vi "GetC.vi"(8 "L1":dbl, 9 "L":dbl, 10 "m":dbl, 11 "q":dbl[](array[numeric])) -> (2 "C":T1)   [LabVIEW 2019]
uses:
  <vilib>/Analysis/Matrix/Datatypes/RealMatrix.ctl
  <vilib>/Analysis/Matrix/NI_Matrix.lvlib
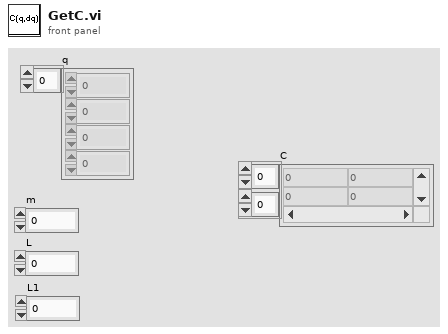
[diagram p1: front panel]
types:
  T1 = typedef "NI_Matrix.lvlib/RealMatrix.ctl" = dbl[][]
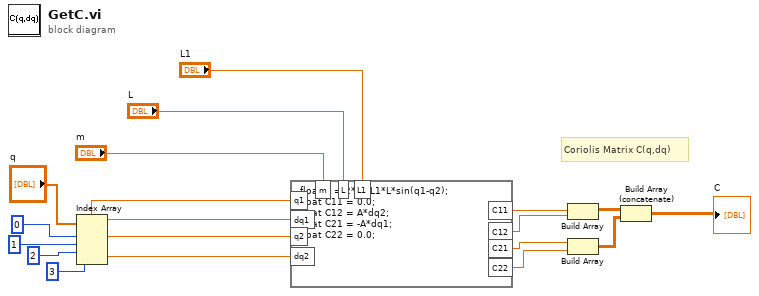
[diagram p0: block diagram]
diagram:
  # "Coriolis Matrix C(q,dq)"
  n1 = Index Array(array="q", index #1=0 ("index (row)"), index #2=1 ("index (col)"), index #3=2 ("index"), index #4=3 ("index")) -> (element #1=w17:dbl, element #2=w13:dbl, element #3=w12:dbl, element #4=w11:dbl)
  n2 = formula code="float A = 2*m*L1*L*sin(q1-q2);\nfloat C11 = 0.0;\nfloat C12 = A*dq2;\nfloat C21 = -A*dq1;\nfloat C22 = 0.0;"("m"="m", "L"="L", "L1"="L1", "q1"=w17, "dq1"=w13, "q2"=w12, "dq2"=w11) -> ("C11"=w4:dbl, "C12"=w3:dbl, "C21"=w2:dbl, "C22"=w1:dbl)
  n3 = Build Array(w4, w3) -> (w7:T1)
  n4 = Build Array(w2, w1) -> (w6:T1)
  n5 = Build Array (concatenate)(w7, w6) -> (→"C":T1)
